vi "Set Channel Units.vi"(8 "error in (no error)":errorcluster, 10 "Units":string, 11 "Channel Reference in":u64 format="%.0x") -> (0 "error out":errorcluster, 3 "Channel Reference out":u64 format="%.0x")   [LabVIEW 2013, in "Hierarchy Framework.lvlib" / "Channel.lvclass"]
doc: "Sets the units of measurement for a channel. <B>Units</B> can be any string that makes sense for your custom device."
uses:
  Channel.lvclass
  Generic/Generic.lvclass
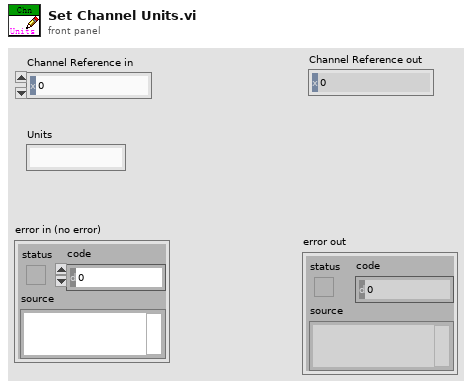
[diagram p1: front panel]
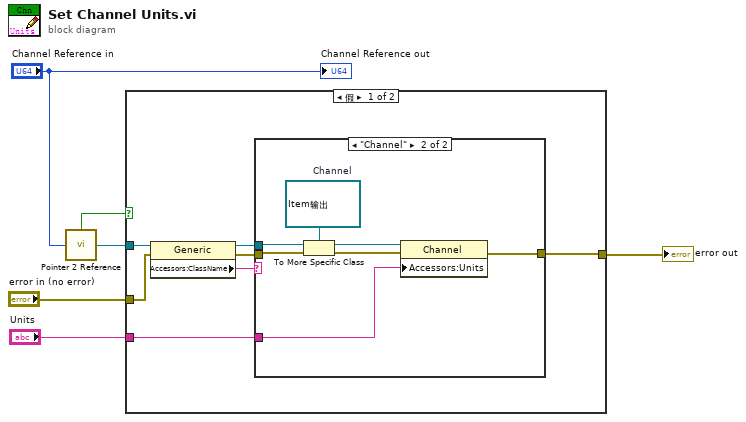
[diagram p0: block diagram]
diagram:
  n1 = call "Pointer 2 Reference.vi"("Pointer"="Channel Reference in") -> ("Not A Refnum?"=w5:bool, "Generic Reference"=w4:refnum<data-value>)
  n2 = case shown="假" w5 {
    tunnel: w4 -> [w13 _]
    tunnel: "error in (no error)" -> [w10 w22]
    tunnel: [w8 w22] -> w2
    tunnel: "Units" -> [w7 _]
    frame False {
      n3 = property class="Generic"(reference=w13, error in=w10) -> (reference out=w11:refnum<data-value>, error out=w9:errorcluster, "Accessors:ClassName"=w12:string)
      n4 = case shown="\"Channel\"" w12 {
        tunnel: w11 -> [_ w21]
        tunnel: w9 -> [w14 w20]
        tunnel: [w14 w16] -> w8
        tunnel: w7 -> [_ w15]
        frame Default {
        }
        frame "Channel" {
          w19 = refnum<data-value> refnum  # Channel
          n5 = To More Specific Class(target class=w19, reference=w21, error in=w20) -> (specific class reference=w18:refnum<data-value>, error out=w17:errorcluster)
          n6 = property class="Channel"(reference=w18, error in=w17, "Accessors:Units"=w15) -> (error out=w16:errorcluster)  [unwired: 1 out]
        }
      }
    }
    frame True {
    }
  }
  "error out" <- w2
  "Channel Reference out" <- "Channel Reference in"
